vi "PH_PILS.Dialog Enabling Warning.vi"() -> (18 "o.k.":bool)   [LabVIEW 2014, in "PH_PILS.lvlib"]
doc: "This VI containes the Warning for the enabling procedure."
uses:
  PH_PILS.lvlib
panel:
  in  "Cancel Button":bool
  in  "OK Button":bool
  # "By pressing ok you are responsible that\nsafe operation is possible and all safety relevant\nadministrative procedures are done."
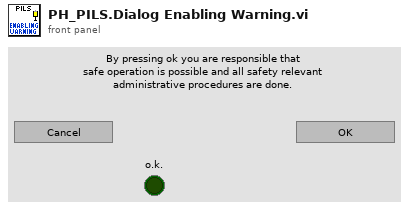
[diagram p1: front panel]
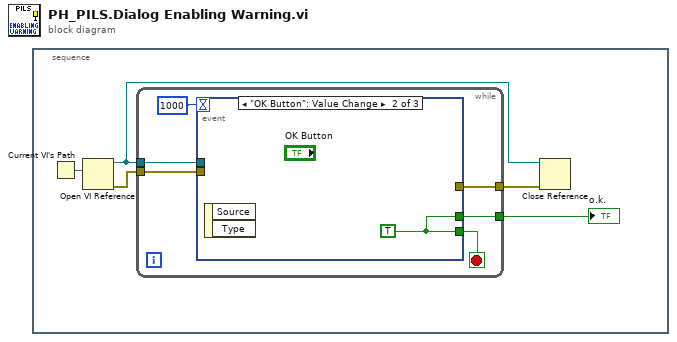
[diagram p0: block diagram]
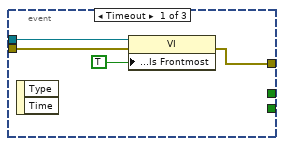
[diagram p2: hidden frame]
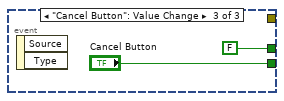
[diagram p3: hidden frame]
diagram:
  n1 = stacked-sequence {
    frame #0 {
      n2 = Current VI's Path() -> (path=w5:path)
      n3 = Open VI Reference(vi path=w5) -> (vi reference=w2:refnum<vi>, error out=w4:errorcluster)  [unwired: 5 in]
      n4 = while {
        tunnel: w2 -> [w10]
        tunnel: w4 -> [w9]
        tunnel: [w8] -> w3
        tunnel: [w6] -> w1
        stop <- w7 stop-if-true
        n5 = event shown="[1] \"OK Button\": Value Change" {
          selector: _ -> [_ _ _]
          dyn-events: _ -> [_ _ _]
          timeout: 1000 -> [_ _ _]
          tunnel: [_ w16 "Cancel Button"] -> w7
          tunnel: w10 -> [w15 _ _]
          tunnel: w9 -> [w14 _ _]
          tunnel: [w12 _ _] -> w8
          tunnel: [_ w16 FALSE] -> w6
          event Timeout {
            n6 = event-data() -> ()  [unwired: 1 in, 2 out]
            n7 = property class="VI"(reference=w15, error in=w14, "Front Panel Window:Is Frontmost"=TRUE) -> (error out=w12:errorcluster)  [unwired: 1 out]
          }
          event "OK Button": Value Change {
            w16 = TRUE
            n8 = event-data() -> ()  [unwired: 1 in, 2 out]
          }
          event "Cancel Button": Value Change {
            n9 = event-data() -> ()  [unwired: 1 in, 2 out]
          }
        }
      }
      "o.k." <- w1
      n10 = Close Reference(reference=w2, error in (no error)=w3) -> ()  [unwired: 1 out]
    }
  }
